vi "Periodic Tasks.vi"(8 "error in (no error)":errorcluster) -> ()   [LabVIEW 2020]
doc: "This VI runs in parallel to other tasks. It can contain as many user-defined periodic loops as you need. These can carry out PID or other sorts of timed response."
uses:
  <vilib>/Rock Robotics/Network Tables/NT Read String.vi
  <vilib>/Rock Robotics/Network Tables/NT Write String.vi
  <vilib>/Rock Robotics/Network Tables/NT Write Number.vi
  Drive/DriveGlobal.vi
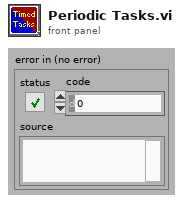
[diagram p1: front panel]
types:
  T1 = typedef "ADIS16470 Device Reference.ctl" = cluster{"DevStatus":errorcluster, "Hardware Config":T2, "Calibration Complete":refnum<notifier>, "Status Reference":refnum<data-value>, "Data Reference":refnum<data-value>, "Sychronous Process VI":T6, "Cmd FIFO":refnum<k33>, "Source":T7, "Data FIFO":refnum<k33>, "Calibration Time (ms)":u32, "Data Reference":refnum<data-value>}
  T2 = typedef "ADIS16470 Hardware Configuration.ctl" = cluster{"SPI Clock Rate (Hz)":dbl, "IMU SPI Mode (3)":T3, "IMU Reset Pin":T4, "IMU SPI Bus":T5, "IMU Data Ready Pin":T4, "Stall Config":cluster{"Pow2BytesPerRead":u8, "StallTicks":u16, "CsToSclkTicks":u8}}
  T3 = typedef "WPI_SPIMode.ctl" = enum16{"Mode 0 (Clk Idle Low,Sample on Leading)", "Mode 1 (Clk Idle Low,Sample on Trailing)", "Mode 2 (Clk Idle High,Sample on Leading)", "Mode 3 (Clk Idle High,Sample on Trailing)"}
  T4 = typedef "FPGA_DIOChannel.ctl" = enum8{"DIO 0", "DIO 1", "DIO 2", "DIO 3", "DIO 4", "DIO 5", "DIO 6", "DIO 7", "DIO 8", "DIO 9", "DIO MXP 0", "DIO MXP 1", "DIO MXP 2", "DIO MXP 3", "DIO MXP 4", "DIO MXP 5", "DIO MXP 6", "DIO MXP 7", "DIO MXP 8", "DIO MXP 9", "DIO MXP 10", "DIO MXP 11", "DIO MXP 12", "DIO MXP 13", "DIO MXP 14", "DIO MXP 15", "SPI Port CS1", "SPI Port CS2", "SPI Port CS3", "SPI Port MISO", "SPI Port MOSI", "Invalid"}
  T5 = typedef "spi_bus.ctl" = enum16{"SPI On-Board, CS0", "SPI On-Board, CS1", "SPI On-Board, CS2", "SPI On-Board, CS3", "SPI MXP", "Invalid"}
  T6 = typedef "ADIS16470 Process.ctl" = refnum<vi>
  T7 = typedef "FPGA_CounterEncoderSourceConvertionLVSourceType.ctl" = cluster{"DevStatus":errorcluster, "AnalogTriggerMode?":bool, "DigitalMode":cluster{"DIO Channel":T8}, "AnalogTriggerMode":cluster{"AnalogTriggerIndex":T9, "OutputType":T10}}
  T8 = typedef "FPGA_DIODigitalSourceChannel.ctl" = enum8{"DIO 0", "DIO 1", "DIO 2", "DIO 3", "DIO 4", "DIO 5", "DIO 6", "DIO 7", "DIO 8", "DIO 9", "DIO MXP 0", "DIO MXP 1", "DIO MXP 2", "DIO MXP 3", "DIO MXP 4", "DIO MXP 5", "DIO MXP 6", "DIO MXP 7", "DIO MXP 8", "DIO MXP 9", "DIO MXP 10", "DIO MXP 11", "DIO MXP 12", "DIO MXP 13", "DIO MXP 14", "DIO MXP 15", "SPI Port CS1", "SPI Port CS2", "SPI Port CS3", "SPI Port MISO", "SPI Port MOSI", "Disabled"}
  T9 = typedef "FPGA_AnalogTriggerIndex.ctl" = enum8{"Trig 0", "Trig 1", "Trig 2", "Trig 3", "Trig 4", "Trig 5", "Trig 6", "Trig 7", "Invalid"}
  T10 = typedef "FPGA_AnalogTriggerOutType.ctl" = enum16{"InWindow", "TriggerState", "Rising", "Falling"}
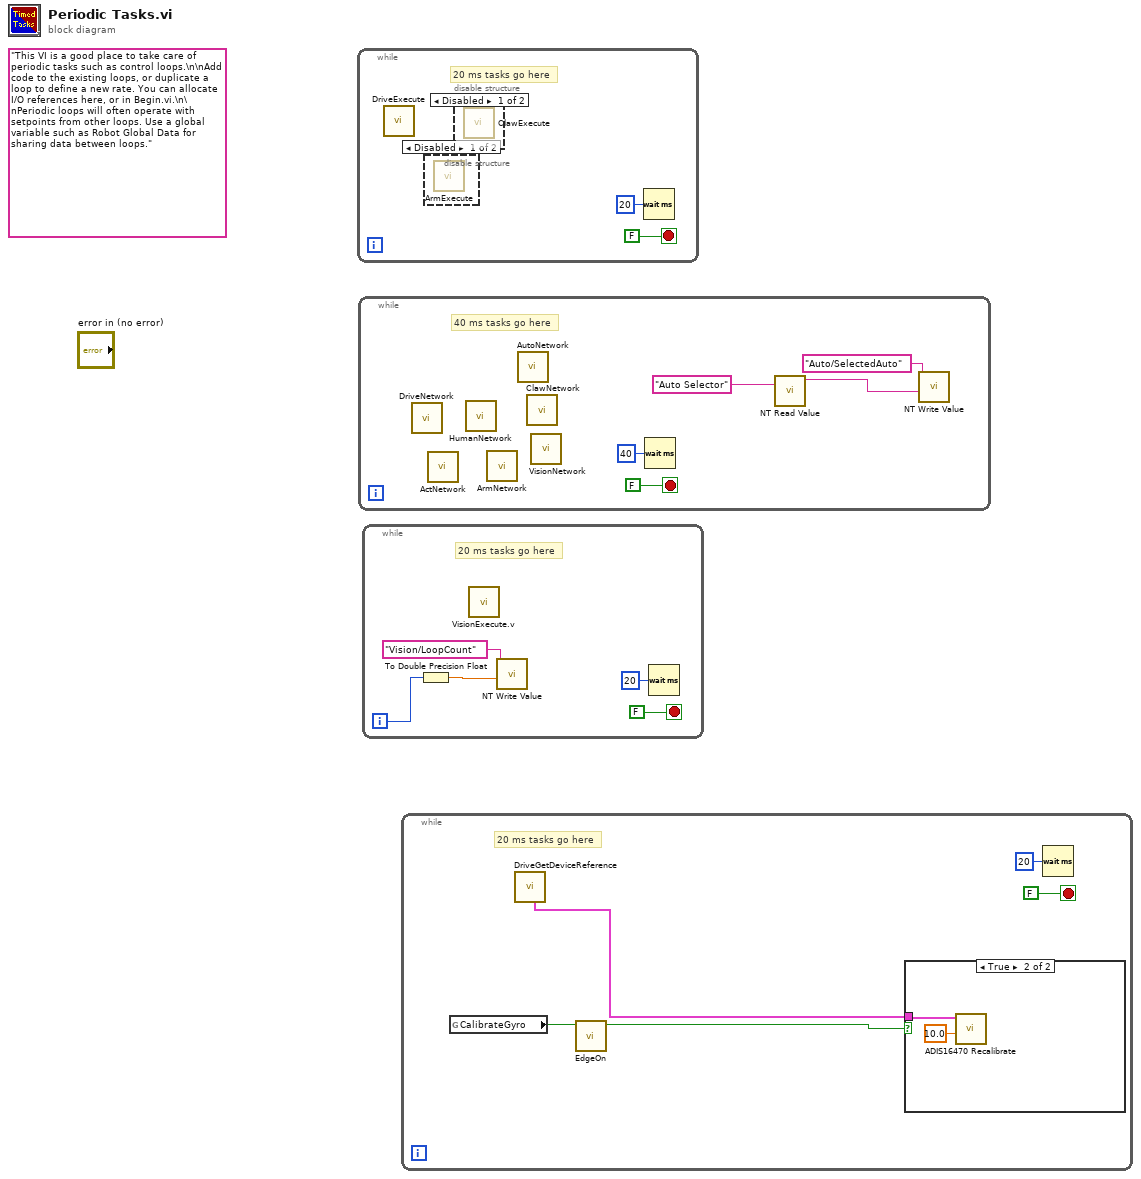
[diagram p0: block diagram]
diagram:
  (unwired) "This VI is a good place to take care of periodic tasks such as control loops.\n\nAdd code to the existing loops, or duplicate a loop to define a new rate. You can allocate I/O references here, or in Begin.vi.\n\nPeriodic loops will often operate with setpoints from other loops. Use a global variable such as Robot Global Data for sharing data between loops."
  n1 = while {
    stop <- FALSE stop-if-true
    # "20 ms tasks go here"
    n2 = call "DriveExecute.vi"() -> ()  [unwired: 11 in, 1 out]
    n3 = disable-structure shown="Disabled" {
      frame Disabled {
        n4 = call "ArmExecute.vi"() -> ()  [unwired: 12 in]
      }
      frame Enabled {
      }
    }
    n5 = disable-structure shown="Disabled" {
      frame Disabled {
        n6 = call "ClawExecute.vi"() -> ()  [unwired: 12 in]
      }
      frame Enabled {
      }
    }
    n7 = Wait (ms)(milliseconds to wait=u32 20) -> ()  [unwired: 1 out]
  }
  n8 = while {
    stop <- FALSE stop-if-true
    # "40 ms tasks go here"
    n9 = call "DriveNetwork.vi"() -> ()  [unwired: 11 in, 1 out]
    n10 = call "ActNetwork.vi"() -> ()  [unwired: 11 in, 1 out]
    n11 = call "HumanNetwork.vi"() -> ()  [unwired: 11 in, 1 out]
    n12 = call "ArmNetwork.vi"() -> ()  [unwired: 11 in, 1 out]
    n13 = call "AutoNetwork.vi"() -> ()  [unwired: 11 in, 1 out]
    n14 = call "ClawNetwork.vi"() -> ()  [unwired: 11 in, 1 out]
    n15 = call "VisionNetwork.vi"() -> ()  [unwired: 11 in, 1 out]
    n16 = Wait (ms)(milliseconds to wait=u32 40) -> ()  [unwired: 1 out]
    n17 = call-poly <vilib>:"NT Read Value.vi"("name"="Auto Selector" ("Name")) -> ("value"=w4:string)  [unwired: 8 in, 2 out]
    n18 = call-poly <vilib>:"NT Write Value.vi"("value"=w4, "name"="Auto/SelectedAuto") -> ()  [unwired: 9 in, 1 out]
  }
  n19 = while {
    i -> [w8]
    stop <- FALSE stop-if-true
    # "20 ms tasks go here"
    n20 = To Double Precision Float(number=w8) -> (double precision float=w9:dbl)
    n21 = call "VisionExecute.v.vi"() -> ()  [unwired: 12 in]
    n22 = call-poly <vilib>:"NT Write Value.vi"("value"=w9, "name"="Vision/LoopCount") -> ()  [unwired: 9 in, 1 out]
    n23 = Wait (ms)(milliseconds to wait=u32 20) -> ()  [unwired: 1 out]
  }
  n24 = while {
    stop <- FALSE stop-if-true
    # "20 ms tasks go here"
    n25 = global read "DriveGlobal.vi" "CalibrateGyro"() -> (w15:bool)
    n26 = call "DriveGetDeviceReference.vi"() -> ("Gryo"=w14:T1)  [unwired: 11 in]
    n27 = call "EdgeOn.vi"("Current State"=w15) -> ("Edge On Found"=w13:bool)  [unwired: 10 in]
    n28 = case shown="True" w13 {
      tunnel: w14 -> [_ w18]
      frame False {
      }
      frame True {
        n29 = call <vilib>:"ADIS16470 Recalibrate.vi"("Calibration Time (4s)"=10.0, "ADIS16470DevRef in"=w18) -> ()  [unwired: 8 in, 2 out]
      }
    }
    n30 = Wait (ms)(milliseconds to wait=u32 20) -> ()  [unwired: 1 out]
  }
